vi "Facade.vi"(0 "Data In":T4, 2 "Display State In":T2, 3 "Container State":T3) -> (6 "Data Out":T4, 7 "Display State Out":T2, 8 "Action":T1)   [LabVIEW 2024, in "Naughty Button.xctl"]
doc: "本VI是为《我和LabVIEW》一书编写的示例。\n关于本书的介绍请参考网页：\nhttp://ruanqizhen.spaces.live.com/blog/cns!5852D4F797C53FB6!4310.entry"
uses:
  Naughty Button.xctl
  Data.ctl
  <vilib>/_xctls/Container State.ctl
  State.ctl
  <vilib>/_xctls/Action.ctl
  <vilib>/_xctls/XControlSupport.lvlib
panel:
  in  "data":bool
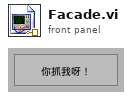
[diagram p1: front panel]
types:
  T1 = typedef "XControlSupport.lvlib/Action.ctl" = cluster{"Data Changed?":bool, "State Changed?":bool, "Action Name":string}
  T2 = typedef "Naughty Button.xctl/State.ctl" = cluster{"Numeric":dbl}
  T3 = typedef "XControlSupport.lvlib/Container State.ctl" = cluster{"Indicator?":bool, "Run Mode?":bool, " Refnum":refnum<vi>}
  T4 = typedef "Naughty Button.xctl/Data.ctl" = bool
  T5 = typedef "LVPositionTypeDef.ctl" = cluster{"Left":i32, "Top":i32}
  T6 = typedef "LVBoundsTypeDef.ctl" = cluster{"Width":u32, "Height":u32}
  T7 = typedef "LVRectTypeDef.ctl" = cluster{"left":i16, "top":i16, "right":i16, "bottom":i16}
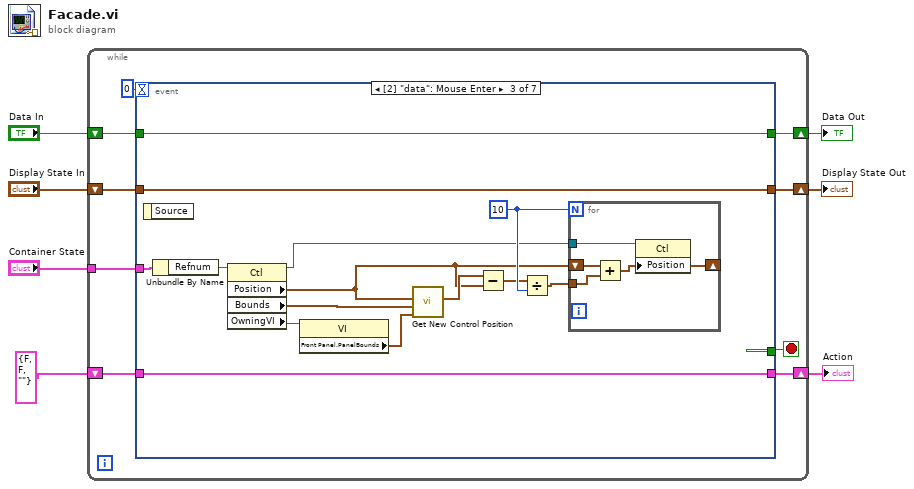
[diagram p0: block diagram]
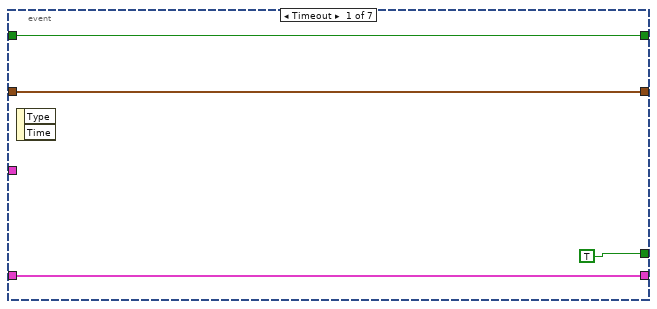
[diagram p2: hidden frame]
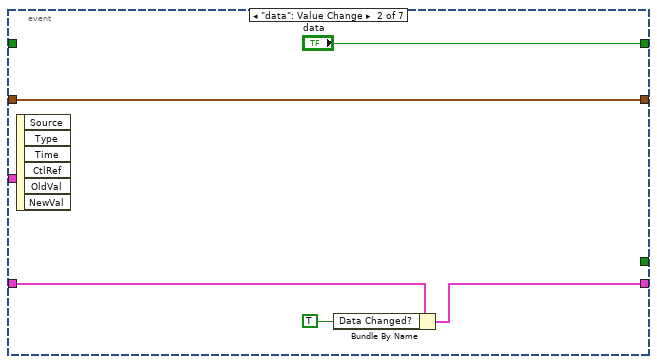
[diagram p3: hidden frame]
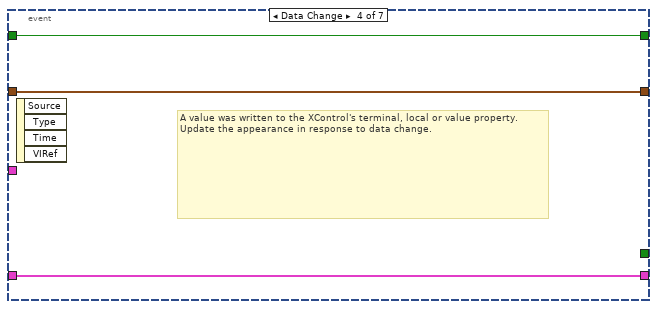
[diagram p4: hidden frame]
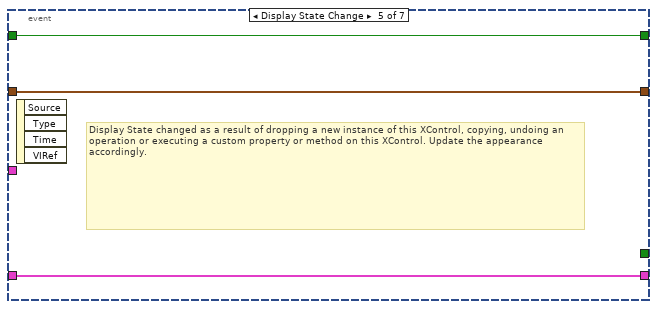
[diagram p5: hidden frame]
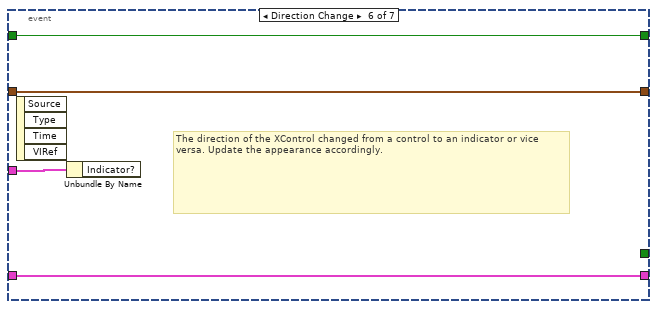
[diagram p6: hidden frame]
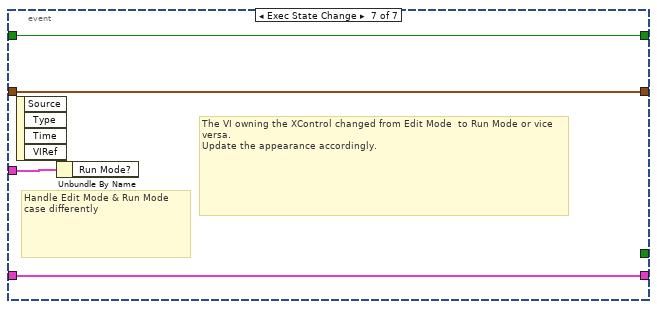
[diagram p7: hidden frame]
diagram:
  n1 = while {
    shift-right: [w15] -> w4
    shift-left: "Display State In" -> [w16]
    tunnel: "Container State" -> [w12]
    shift-right: [w10] -> w7
    shift-left: "Data In" -> [w11]
    shift-right: [w8] -> w2
    shift-left: T1 {"Data Changed?"=FALSE, "State Changed?"=FALSE, "Action Name"=""} ("Action") -> [w9]
    stop <- w14 stop-if-true
    n2 = event shown="[2] \"data\": Mouse Enter" {
      selector: _ -> [_ _ _ _ _ _ _]
      dyn-events: _ -> [_ _ _ _ _ _ _]
      timeout: 0 -> [_ _ _ _ _ _ _]
      tunnel: w16 -> [w19 w24 w39 w45 w49 w52 w56]
      tunnel: [w19 w24 w39 w45 w49 w52 w56] -> w15
      tunnel: [TRUE _ _ _ _ _ _] -> w14
      tunnel: w12 -> [_ _ w35 _ _ w53 w57]
      tunnel: w11 -> [w18 _ w38 w46 w48 w51 w55]
      tunnel: [w18 "data" w38 w46 w48 w51 w55] -> w10
      tunnel: [w17 w21 w37 w44 w47 w50 w54] -> w8
      tunnel: w9 -> [w17 w23 w37 w44 w47 w50 w54]
      event Timeout {
        n3 = event-data() -> ()  [unwired: 3 out]
      }
      event "data": Value Change {
        n4 = event-data() -> ()  [unwired: 7 out]
        n5 = Bundle By Name(cluster=w23, "Data Changed?"=TRUE) -> (w21:T1)
      }
      event "data": Mouse Enter {
        w31 = 10
        n6 = event-data() -> ()  [unwired: 2 out]
        n7 = Unbundle By Name(w35) -> ("Refnum"=w36:refnum<vi>)
        n8 = property class="Ctl"(reference=w36) -> (reference out=w26:refnum<vi>, "Position"=w28:T5, "Bounds"=w33:T6, "OwningVI"=w34:refnum<vi>)  [unwired: 1 in, 1 out]
        n9 = property class="VI"(reference=w34) -> ("Front Panel.PanelBounds"=w32:T7)  [unwired: 1 in, 2 out]
        n10 = call "Get New Control Position.vi"("panel bounds"=w32, "边界"=w33, "位置"=w28) -> ("位置"=w29:T5)  [unwired: 8 out]
        n11 = Subtract(x=w29, y=w28) -> (x-y=w27:T5)
        n12 = Divide(x=w27, y=w31) -> (x/y=w30:cluster{"Left":dbl, "Top":dbl})
        n13 = for {
          N: w31 -> [_]
          tunnel: w26 -> [w43]
          shift-right: [w40] -> _
          shift-left: w28 -> [w42]
          tunnel: w30 -> [w41]
          n14 = Add(x=w42, y=w41) -> (x+y=w40:cluster{"Left":dbl, "Top":dbl})
          n15 = property class="Ctl"(reference=w43, "Position"=w40) -> ()  [unwired: 1 in, 2 out]
        }
      }
      event Data Change {
        # "A value was written to the XControl's terminal, local or value property.\nUpdate the appearance in response to data change."
        n16 = event-data() -> ()  [unwired: 5 out]
      }
      event Display State Change {
        # "Display State changed as a result of dropping a new instance of this XControl, copying, undoing an operation or executing a custom property or method on this XControl. Update the appearance accordingly."
        n17 = event-data() -> ()  [unwired: 5 out]
      }
      event Direction Change {
        # "The direction of the XControl changed from a control to an indicator or vice versa. Update the appearance accordingly."
        n18 = event-data() -> ()  [unwired: 5 out]
        n19 = Unbundle By Name(w53) -> ()  [unwired: 1 out]
      }
      event Exec State Change {
        # "The VI owning the XControl changed from Edit Mode  to Run Mode or vice versa.\nUpdate the appearance accordingly."
        # "Handle Edit Mode & Run Mode\ncase differently"
        n20 = event-data() -> ()  [unwired: 5 out]
        n21 = Unbundle By Name(w57) -> ()  [unwired: 1 out]
      }
    }
  }
  "Display State Out" <- w4
  "Data Out" <- w7
  "Action" <- w2
